vi "Convert Genealogy to Binary.vi"(8 "error in (no error)":errorcluster, 10 "SN In":string="QMC2200123", 11 "PN In":string="10-000001") -> (0 "error out":errorcluster, 1 "week and serial (32bit) out":i32, 2 "Vendor (8bit) out":u8[](array[numeric]), 3 "PN 64Base out":u8[](array[numeric]))   [LabVIEW 2021, in "CAN wrapper.lvlib"]
uses:
  CAN wrapper.lvlib
panel:
  # "e.g. QMC2200123"
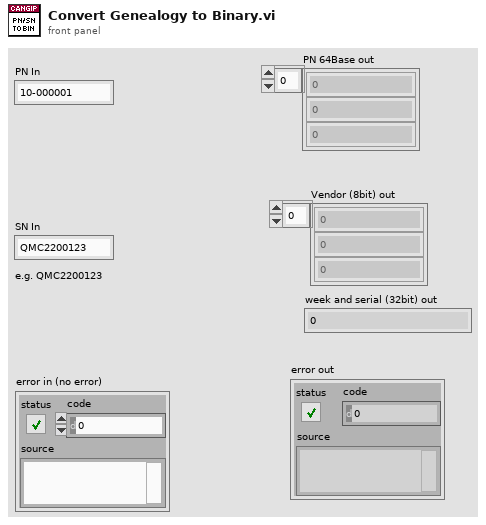
[diagram p1: front panel]
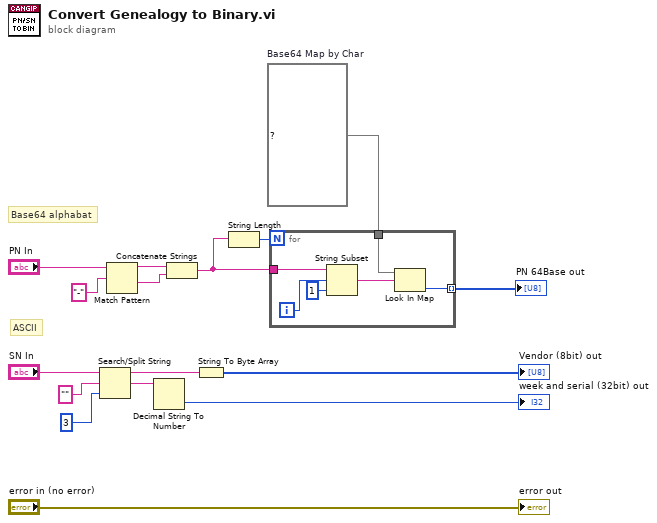
[diagram p0: block diagram]
diagram:
  w3 = map{string, u8} {"+"=62, "/"=63, "0"=52, "1"=53, "2"=54, "3"=55, "4"=56, "5"=57, "6"=58, "7"=59, "8"=60, "9"=61, "A"=0, "B"=1, "C"=2, "D"=3, "E"=4, "F"=5, "G"=6, "H"=7, "I"=8, "J"=9, "K"=10, "L"=11, "M"=12, "N"=13, "O"=14, "P"=15, "Q"=16, "R"=17, "S"=18, "T"=19, "U"=20, "V"=21, "W"=22, "X"=23, "Y"=24, "Z"=25, "a"=26, "b"=27, "c"=28, "d"=29, "e"=30, "f"=31, "g"=32, "h"=33, "i"=34, "j"=35, "k"=36, "l"=37, "m"=38, "n"=39, "o"=40, "p"=41, "q"=42, "r"=43, "s"=44, "t"=45, "u"=46, "v"=47, "w"=48, "x"=49, "y"=50, "z"=51}  # Base64 Map by Char
  # "ASCII"
  # "Base64 alphabat"
  n1 = Search/Split String(string="SN In", search string/char (-)="", offset (0)=3) -> (substring before match=w13:string, match + rest of string=w12:string)  [unwired: 1 out]
  n2 = Match Pattern(string="PN In", regular expression="-") -> (before substring=w6:string, after substring=w5:string)  [unwired: 1 in, 2 out]
  n3 = Decimal String To Number(string=w12) -> (number=→"week and serial (32bit) out":i32)  [unwired: 2 in, 1 out]
  n4 = Concatenate Strings(w6, w5) -> (w2:string)
  n5 = String To Byte Array(string=w13) -> (unsigned byte array=→"Vendor (8bit) out":u8[])
  n6 = String Length(string=w2) -> (length=w4:i32)
  n7 = for {
    N: w4 -> [_]
    tunnel: w2 -> [w21]
    tunnel: w3 -> [w18]
    tunnel: [w17] -> w1 mode=indexing
    i -> [w20]
    n8 = String Subset(string=w21, offset (0)=w20, length (rest)=1 ("length (rest)")) -> (substring=w19:string)
    n9 = Look In Map(map=w18, key=w19) -> (value=w17:u8)  [unwired: 1 in, 1 out]
  }
  "PN 64Base out" <- w1
  "error out" <- "error in (no error)"
